vi "Parse Config Query Resp.vi"(8 "error in":errorcluster, 10 "State":string, 11 "Kronos in":refnum<class "Kronos.lvclass">) -> (0 "error out":errorcluster, 3 "Kronos out":refnum<class "Kronos.lvclass">)   [LabVIEW 2018, in "Kronos.lvlib" / "Kronos.lvclass"]
uses:
  Kronos.lvclass
  builds/Laser.lvlibp/Laser.lvclass
  C:/Users/Ron.Dexter.LUMINARTECH/Desktop/builds/Laser.lvlibp/Laser.lvclass
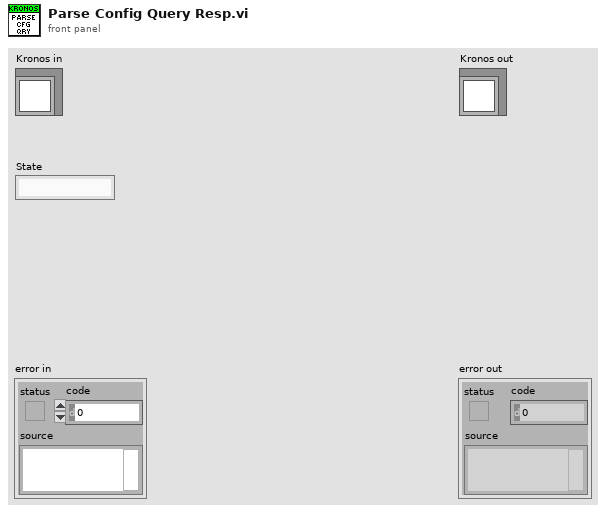
[diagram p1: front panel]
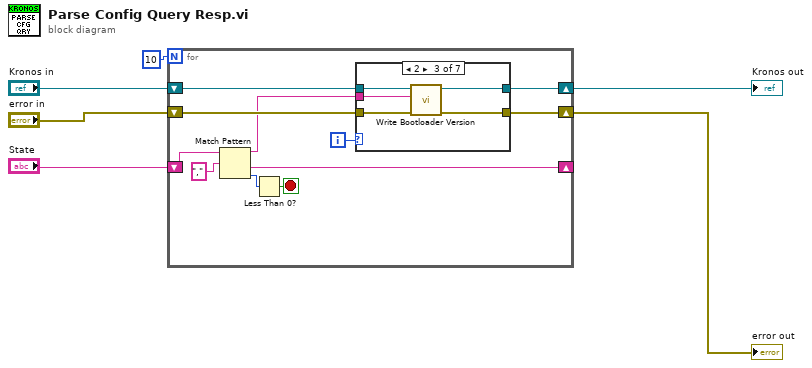
[diagram p0: block diagram]
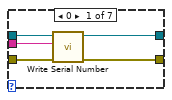
[diagram p2: hidden frame]
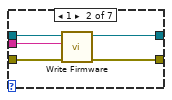
[diagram p3: hidden frame]
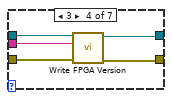
[diagram p4: hidden frame]
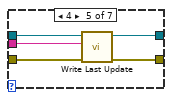
[diagram p5: hidden frame]
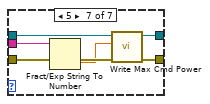
[diagram p7: hidden frame]
diagram:
  n1 = for {
    N: 10 -> [_]
    shift-right: [w16] -> _
    shift-left: "State" -> [w17]
    shift-right: [w9] -> w2
    shift-left: "Kronos in" -> [w11]
    shift-right: [w8] -> w1
    shift-left: "error in" -> [w10]
    i -> [w12]
    stop <- w13 stop-if-true
    n2 = Match Pattern(string=w17, regular expression=",") -> (before substring=w7:string, after substring=w16:string, offset past match=w14:i32)  [unwired: 1 in, 1 out]
    n3 = Less Than 0?(x=w14) -> (x < 0?=w13:bool)
    n4 = case shown="2" w12 {
      tunnel: w11 -> [w21 w27 w32 w37 w42 w43 w50]
      tunnel: w10 -> [w22 w26 w30 w35 w40 w44 w47]
      tunnel: [w20 w24 w31 w33 w38 w43 w49] -> w9
      tunnel: [w19 w23 w29 w34 w39 w44 w48] -> w8
      tunnel: w7 -> [w18 w25 w28 w36 w41 _ w46]
      frame 0 {
        n5 = call "Write Serial Number.vi"("error in (no error)"=w22, "Serial Number"=w18, "Laser in"=w21) -> ("error out"=w19:errorcluster, "Laser out"=w20:refnum<class "Kronos.lvclass">)  [unwired: 7 in]
      }
      frame 1 {
        n6 = call "Write Firmware.vi"("error in (no error)"=w26, "Firmware"=w25, "Laser in"=w27) -> ("error out"=w23:errorcluster, "Laser out"=w24:refnum<class "Kronos.lvclass">)  [unwired: 7 in]
      }
      frame 2 {
        n7 = call "Write Bootloader Version.vi"("error in (no error)"=w30, "Bootloader Version"=w28, "Laser in"=w32) -> ("error out"=w29:errorcluster, "Laser out"=w31:refnum<class "Kronos.lvclass">)  [unwired: 7 in]
      }
      frame 3 {
        n8 = call "Write FPGA Version.vi"("error in (no error)"=w35, "FPGA Version"=w36, "Laser in"=w37) -> ("error out"=w34:errorcluster, "Laser out"=w33:refnum<class "Kronos.lvclass">)  [unwired: 7 in]
      }
      frame 4 {
        n9 = call "Write Last Update.vi"("error in (no error)"=w40, "Last Update"=w41, "Laser in"=w42) -> ("error out"=w39:errorcluster, "Laser out"=w38:refnum<class "Kronos.lvclass">)  [unwired: 7 in]
      }
      frame Default {
      }
      frame 5 {
        n10 = Fract/Exp String To Number(string=w46) -> (number=w45:dbl)  [unwired: 3 in, 1 out]
        n11 = call "Write Max Cmd Power.vi"("error in (no error)"=w47, "Max Cmd Power"=w45, "Laser in"=w50) -> ("error out"=w48:errorcluster, "Laser out"=w49:refnum<class "Kronos.lvclass">)  [unwired: 7 in]
      }
    }
  }
  "error out" <- w1
  "Kronos out" <- w2
